vi "Create Env Internal.vi"(8 "error in (no error)":errorcluster, 10 "?":T2, 11 "Paths":T1) -> (0 "error out":errorcluster, 3 "Env":refnum<k24>)   [LabVIEW 2020, in "WebView2.lvlib" / "WebView2 Control.lvclass"]
uses:
  WebView2 Control.lvclass
  C:/Users/Simon/Documents/GitHub/LV-WebView2/Source/Libs/Microsoft.Web.WebView2.Core.dll
  Libs/Microsoft.Web.WebView2.Core.dll
  WebView2 Control.lvclass/WebView2 Control.ctl
  Core Env Options.ctl
  Paths.ctl
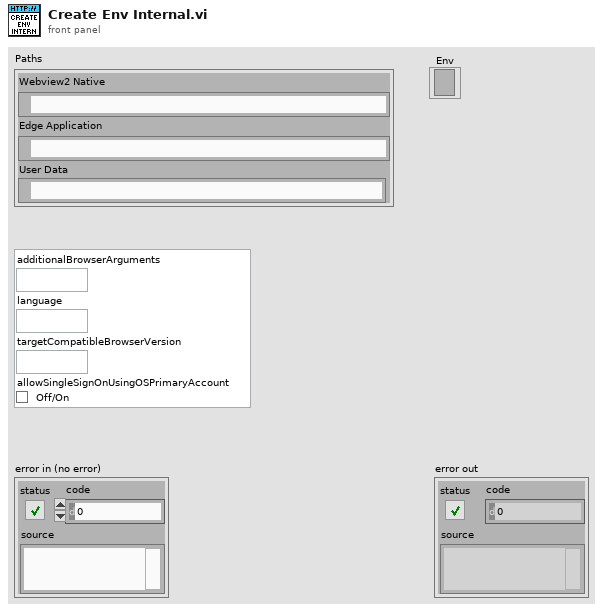
[diagram p1: front panel]
types:
  T1 = typedef "WebView2.lvlib/WebView2 Control.lvclass/Paths.ctl" = cluster{"Webview2 Native":path, "Edge Application":path, "User Data":path}
  T2 = typedef "WebView2.lvlib/WebView2 Control.lvclass/Core Env Options.ctl" = cluster{"additionalBrowserArguments":string, "language":string, "targetCompatibleBrowserVersion":string, "allowSingleSignOnUsingOSPrimaryAccount":bool}
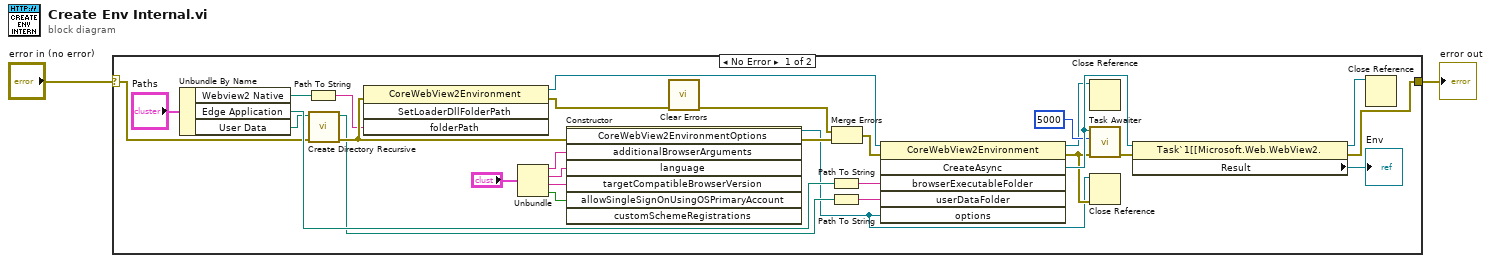
[diagram p0: block diagram]
diagram:
  n1 = case shown="No Error" "error in (no error)" {
    selector: "error in (no error)" -> [w7 w32]
    tunnel: [w22 w32] -> w2
    frame No Error {
      n2 = Unbundle By Name("Paths") -> ("Webview2 Native"=w29:path, "Edge Application"=w31:path, "User Data"=w30:path)
      n3 = Path To String(path=w29) -> (string=w18:string)
      n4 = call <vilib>:"Create Directory Recursive.vi"("error in (no error)"=w7, "directory"=w30) -> ("error out"=w19:errorcluster, "directory copy"=w16:path)  [unwired: 3 in, 1 out]
      n5 = invoke class="CoreWebView2Environment" method="SetLoaderDllFolderPath"(error in=w19, "folderPath"=w18) -> (reference out=w5:refnum<k24>, error out=w4:errorcluster)  [unwired: 2 in, 2 out]
      n6 = Unbundle("?") -> ("additionalBrowserArguments"=w10:string, "language"=w11:string, "targetCompatibleBrowserVersion"=w12:string, "allowSingleSignOnUsingOSPrimaryAccount"=w13:bool)
      n7 = constructor class="CoreWebView2EnvironmentOptions"(error in=w19, "additionalBrowserArguments"=w10, "language"=w11, "targetCompatibleBrowserVersion"=w12, "allowSingleSignOnUsingOSPrimaryAccount"=w13) -> (reference out=w14:refnum<k24>, error out=w15:errorcluster)  [unwired: 3 in, 6 out]
      n8 = call <vilib>:"Clear Errors.vi"("error in (no error)"=w4) -> ("error out"=w3:errorcluster)  [unwired: 5 in, 1 out]
      n9 = Path To String(path=w31) -> (string=w6:string)
      n10 = Path To String(path=w16) -> (string=w17:string)
      n11 = Merge Errors(w3, w15) -> (w23:errorcluster)
      n12 = invoke class="CoreWebView2Environment" method="CreateAsync"(reference=w5, error in=w23, "browserExecutableFolder"=w6, "userDataFolder"=w17, "options"=w14) -> (reference out=w8:refnum<k24>, error out=w20:errorcluster, "CreateAsync"=w26:refnum<k24>)  [unwired: 1 in, 3 out]
      n13 = Close Reference(reference=w8) -> ()  [unwired: 1 in, 1 out]
      n14 = call "Task Awaiter.vi"("error in (no error)"=w20, "Timeout"=5000 ("millisecondsTimeout"), "Task"=w26) -> ("error out"=w24:errorcluster)  [unwired: 6 in, 2 out]
      n15 = Close Reference(reference=w14, error in (no error)=w20) -> ()  [unwired: 1 out]
      n16 = property class="Task`1[[Microsoft.Web.WebView2."(reference=w26, error in=w24) -> (reference out=w21:refnum<k24>, error out=w22:errorcluster, "Result"=→"Env":refnum<k24>)
      n17 = Close Reference(reference=w21) -> ()  [unwired: 1 in, 1 out]
    }
    frame Error {
    }
  }
  "error out" <- w2
